vi "simple for.vi"() -> ()   [LabVIEW 2020]
uses:
  point.ctl
panel:
  out "target Point":T1
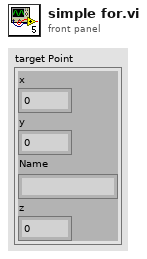
[diagram p1: front panel]
types:
  T1 = typedef "point.ctl" = cluster{"x":i32, "y":i32, "Name":string, "z":i32}
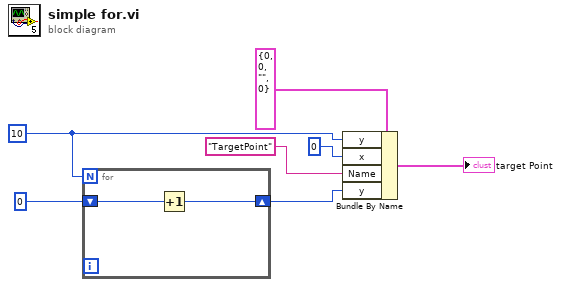
[diagram p0: block diagram]
diagram:
  w5 = 10
  n1 = for {
    N: w5 -> [_]
    shift-right: [w9] -> w4
    shift-left: 0 -> [w8]
    n2 = Increment(x=w8) -> (x+1=w9:i32)
  }
  n3 = Bundle By Name(cluster=T1 {"x"=0, "y"=0, "Name"="", "z"=0}, "y"=w5, "x"=0 ("y"), "Name"="TargetPoint", "y"=w4) -> (→"target Point":T1)
